vi "hamilton_controller.vi"(8 "error in":errorcluster, 9 "Open?":bool, 10 "valve":enum16{"A", "B", "C", "D", "ALL"}(ring), 11 "action":T1(ring)) -> (0 "error out":errorcluster)   [LabVIEW 2014]
uses:
  <vilib>/Instr/_visa.llb/VISA Configure Serial Port (Instr).vi
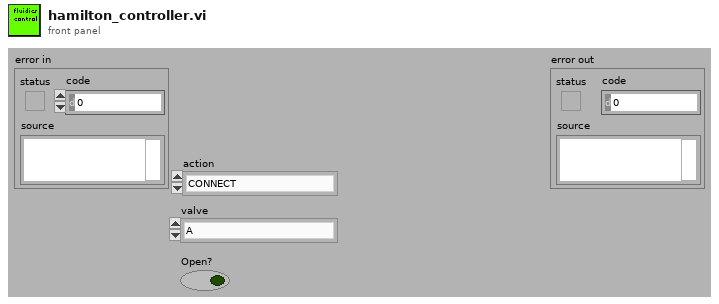
[diagram p1: front panel]
types:
  T1 = enum16{"CONNECT", "INITIALIZE VALVES", "DISCONNECT", "MOVE VALVE"}
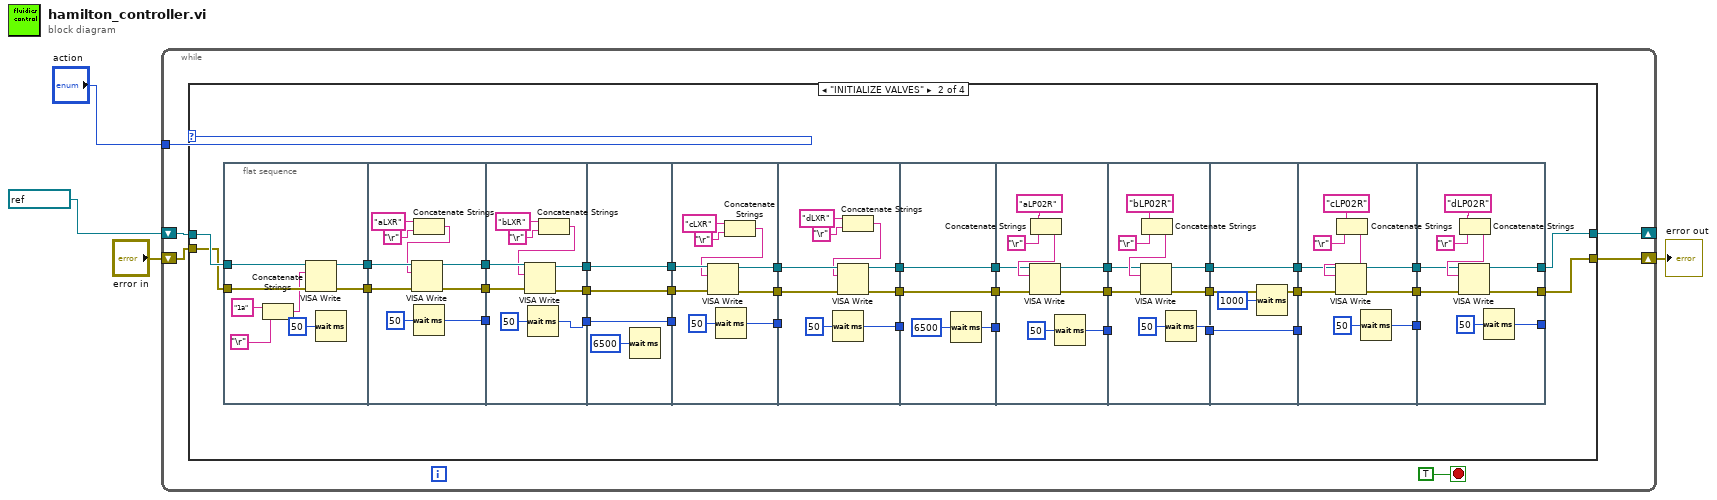
[diagram p0: block diagram]
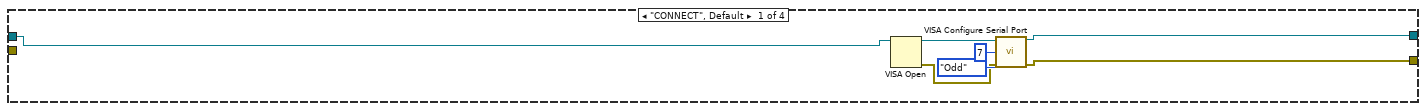
[diagram p2: hidden frame]
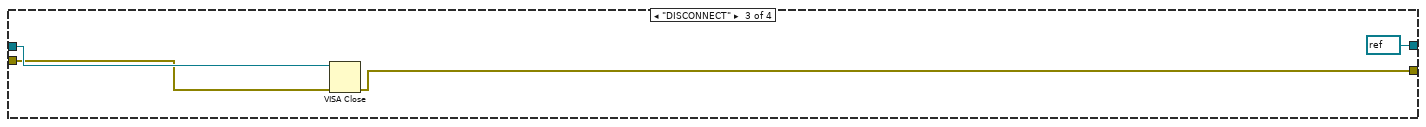
[diagram p3: hidden frame]
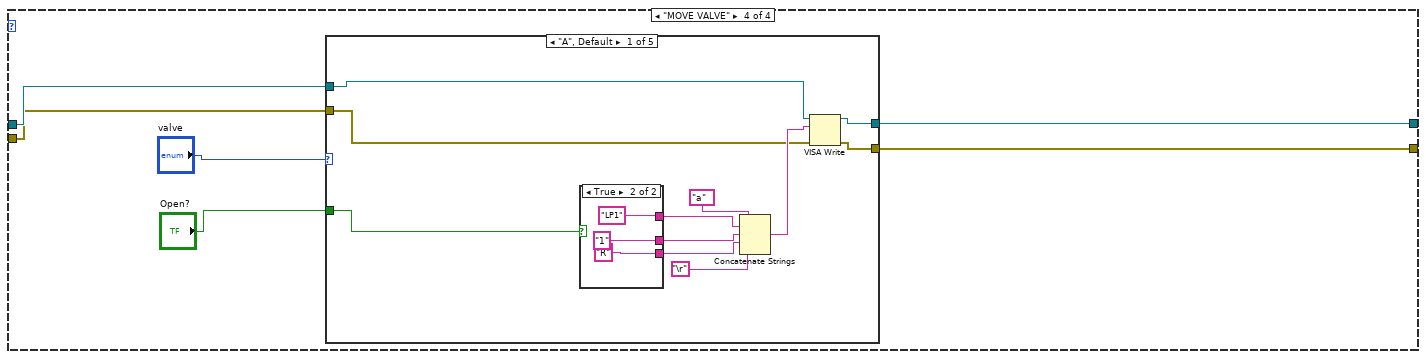
[diagram p4: hidden frame]
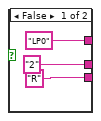
[diagram p5: hidden frame]
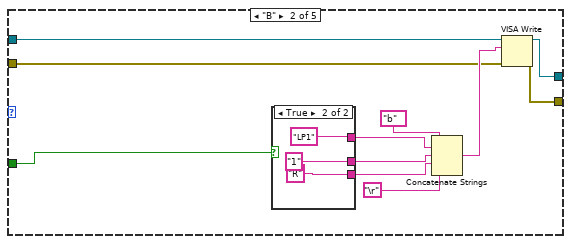
[diagram p6: hidden frame]
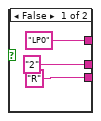
[diagram p7: hidden frame]
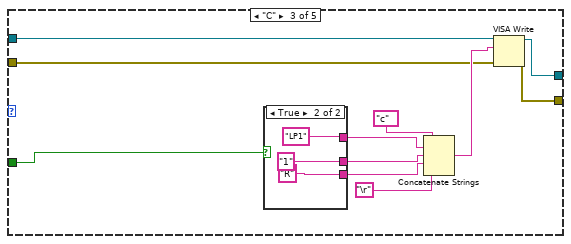
[diagram p8: hidden frame]
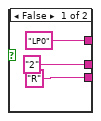
[diagram p9: hidden frame]
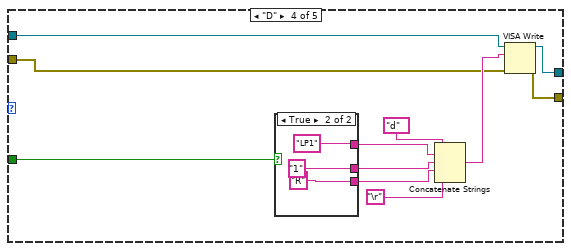
[diagram p10: hidden frame]
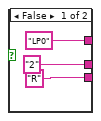
[diagram p11: hidden frame]
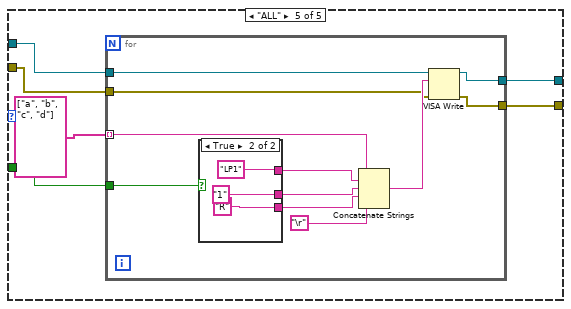
[diagram p12: hidden frame]
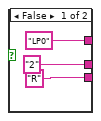
[diagram p13: hidden frame]
diagram:
  n1 = while {
    tunnel: "action" -> [w9]
    shift-right: [w8] -> _
    shift-left: refnum<visa-resource-name> "COM6" ("VISA resource name") -> [w6]
    shift-right: [w7] -> w2
    shift-left: "error in" -> [w5]
    stop <- TRUE stop-if-true
    n2 = case shown="\"INITIALIZE VALVES\"" w9 {
      tunnel: [w13 w19 refnum<visa-resource-name> refnum ("VISA resource name out") w152] -> w8
      tunnel: [w12 w18 w147 w151] -> w7
      tunnel: w6 -> [w11 w21 w149 w154]
      tunnel: w5 -> [_ w20 w148 w153]
      frame "CONNECT", Default {
        n3 = VISA Open(VISA resource name=w11) -> (VISA resource name=w17:refnum<visa-resource-name>, error out=w14:errorcluster)  [unwired: 4 in]
        n4 = call-poly "VISA Configure Serial Port"("VISA resource name"=w17, "data bits (8)"=u16 7, "parity (0:none)"=enum16{"None", "Odd", "Even", "Mark", "Space"}."Odd", "error in (no error)"=w14) -> ("VISA resource name out"=w13:refnum<visa-resource-name>, "error out"=w12:errorcluster)  [unwired: 10 in]
      }
      frame "INITIALIZE VALVES" {
        n5 = flat-sequence {
          tunnel: w21 -> [w61]
          tunnel: w20 -> [w60]
          tunnel: [w59] -> w53
          tunnel: [w55] -> w52
          tunnel: w53 -> [w69]
          tunnel: w52 -> [w70]
          tunnel: [w68] -> w51
          tunnel: [w63] -> w50
          tunnel: [w62] -> w49
          tunnel: w51 -> [_]
          tunnel: w50 -> [w79]
          tunnel: [w78] -> w48
          tunnel: w49 -> [w77]
          tunnel: [w76] -> w47
          tunnel: [w74] -> w46
          tunnel: w48 -> [w83]
          tunnel: [w83] -> w45
          tunnel: w47 -> [w82]
          tunnel: [w82] -> w44
          tunnel: w46 -> [w81]
          tunnel: [w81] -> w43
          tunnel: w45 -> [w92]
          tunnel: [w91] -> w42
          tunnel: w44 -> [w90]
          tunnel: [w89] -> w41
          tunnel: w43 -> [_]
          tunnel: [w87] -> w40
          tunnel: w42 -> [w101]
          tunnel: w41 -> [w100]
          tunnel: w40 -> [_]
          tunnel: [w95] -> w39
          tunnel: [w94] -> w38
          tunnel: [w93] -> w37
          tunnel: w39 -> [w102]
          tunnel: w38 -> [w105]
          tunnel: [w105] -> w36
          tunnel: w37 -> [_]
          tunnel: [w103] -> w35
          tunnel: [w102] -> w34
          tunnel: w36 -> [w108]
          tunnel: w35 -> [_]
          tunnel: w34 -> [w106]
          tunnel: [w111] -> w33
          tunnel: [w109] -> w32
          tunnel: [w107] -> w31
          tunnel: w33 -> [w118]
          tunnel: w32 -> [_]
          tunnel: [w117] -> w30
          tunnel: [w119] -> w29
          tunnel: w31 -> [w116]
          tunnel: [w115] -> w28
          tunnel: w30 -> [w127]
          tunnel: [w127] -> w27
          tunnel: w29 -> [w126]
          tunnel: [w126] -> w26
          tunnel: w28 -> [w125]
          tunnel: [w125] -> w25
          tunnel: w27 -> [w131]
          tunnel: w26 -> [_]
          tunnel: [w132] -> w24
          tunnel: [w130] -> w23
          tunnel: w25 -> [w129]
          tunnel: [w128] -> w22
          tunnel: w24 -> [_]
          tunnel: [w141] -> _
          tunnel: w23 -> [w140]
          tunnel: [w139] -> w18
          tunnel: w22 -> [w138]
          tunnel: [w137] -> w19
          frame #0 {
            n6 = Concatenate Strings("1a" ("string"), "\r") -> (w56:string)
            n7 = VISA Write(VISA resource name=w61, write buffer=w56, error in (no error)=w60) -> (VISA resource name out=w55:refnum<visa-resource-name>, error out=w59:errorcluster)  [unwired: 1 out]
            n8 = Wait (ms)(milliseconds to wait=u32 50) -> ()  [unwired: 1 out]
          }
          frame #1 {
            n9 = Concatenate Strings("aLXR", "\r") -> (w64:string)
            n10 = VISA Write(VISA resource name=w70, write buffer=w64, error in (no error)=w69) -> (VISA resource name out=w63:refnum<visa-resource-name>, error out=w62:errorcluster)  [unwired: 1 out]
            n11 = Wait (ms)(milliseconds to wait=u32 50) -> (millisecond timer value=w68:u32)
          }
          frame #2 {
            n12 = Wait (ms)(milliseconds to wait=u32 50) -> (millisecond timer value=w74:u32)
            n13 = Concatenate Strings("bLXR", "\r") -> (w71:string)
            n14 = VISA Write(VISA resource name=w79, write buffer=w71, error in (no error)=w77) -> (VISA resource name out=w78:refnum<visa-resource-name>, error out=w76:errorcluster)  [unwired: 1 out]
          }
          frame #3 {
            n15 = Wait (ms)(milliseconds to wait=u32 6500) -> ()  [unwired: 1 out]
          }
          frame #4 {
            n16 = Wait (ms)(milliseconds to wait=u32 50) -> (millisecond timer value=w87:u32)
            n17 = Concatenate Strings("cLXR", "\r") -> (w84:string)
            n18 = VISA Write(VISA resource name=w92, write buffer=w84, error in (no error)=w90) -> (VISA resource name out=w91:refnum<visa-resource-name>, error out=w89:errorcluster)  [unwired: 1 out]
          }
          frame #5 {
            n19 = Wait (ms)(milliseconds to wait=u32 50) -> (millisecond timer value=w93:u32)
            n20 = Concatenate Strings("dLXR", "\r") -> (w96:string)
            n21 = VISA Write(VISA resource name=w101, write buffer=w96, error in (no error)=w100) -> (VISA resource name out=w94:refnum<visa-resource-name>, error out=w95:errorcluster)  [unwired: 1 out]
          }
          frame #6 {
            n22 = Wait (ms)(milliseconds to wait=u32 6500) -> (millisecond timer value=w103:u32)
          }
          frame #7 {
            n23 = Concatenate Strings("aLP02R" ("string"), "\r") -> (w114:string)
            n24 = VISA Write(VISA resource name=w108, write buffer=w114, error in (no error)=w106) -> (VISA resource name out=w107:refnum<visa-resource-name>, error out=w111:errorcluster)  [unwired: 1 out]
            n25 = Wait (ms)(milliseconds to wait=u32 50) -> (millisecond timer value=w109:u32)
          }
          frame #8 {
            n26 = Concatenate Strings("bLP02R" ("string"), "\r") -> (w123:string)
            n27 = VISA Write(VISA resource name=w116, write buffer=w123, error in (no error)=w118) -> (VISA resource name out=w115:refnum<visa-resource-name>, error out=w117:errorcluster)  [unwired: 1 out]
            n28 = Wait (ms)(milliseconds to wait=u32 50) -> (millisecond timer value=w119:u32)
          }
          frame #9 {
            n29 = Wait (ms)(milliseconds to wait=u32 1000) -> ()  [unwired: 1 out]
          }
          frame #10 {
            n30 = Concatenate Strings("cLP02R" ("string"), "\r") -> (w136:string)
            n31 = VISA Write(VISA resource name=w129, write buffer=w136, error in (no error)=w131) -> (VISA resource name out=w128:refnum<visa-resource-name>, error out=w130:errorcluster)  [unwired: 1 out]
            n32 = Wait (ms)(milliseconds to wait=u32 50) -> (millisecond timer value=w132:u32)
          }
          frame #11 {
            n33 = Concatenate Strings("dLP02R" ("string"), "\r") -> (w145:string)
            n34 = VISA Write(VISA resource name=w138, write buffer=w145, error in (no error)=w140) -> (VISA resource name out=w137:refnum<visa-resource-name>, error out=w139:errorcluster)  [unwired: 1 out]
            n35 = Wait (ms)(milliseconds to wait=u32 50) -> (millisecond timer value=w141:u32)
          }
        }
      }
      frame "DISCONNECT" {
        n36 = VISA Close(VISA resource name=w149, error in (no error)=w148) -> (error out=w147:errorcluster)
      }
      frame "MOVE VALVE" {
        n37 = case shown="\"A\", Default" "valve" {
          tunnel: w154 -> [w160 w177 w192 w211 w229]
          tunnel: w153 -> [w159 w176 w191 w210 w226]
          tunnel: [w158 w175 w194 w209 w224] -> w152
          tunnel: [w157 w174 w193 w208 w225] -> w151
          tunnel: "Open?" -> [w156 w173 w190 w207 w228]
          frame "A", Default {
            n38 = case shown="True" w156 {
              tunnel: ["R" "R"] -> w164
              tunnel: ["2" "1"] -> w165
              tunnel: ["LP0" ("string") "LP1" ("string")] -> w162
              frame False {
              }
              frame True {
              }
            }
            n39 = Concatenate Strings("a" ("MVP ID"), w162, w165, w164, "\r") -> (w161:string)
            n40 = VISA Write(VISA resource name=w160, write buffer=w161, error in (no error)=w159) -> (VISA resource name out=w158:refnum<visa-resource-name>, error out=w157:errorcluster)  [unwired: 1 out]
          }
          frame "B" {
            n41 = case shown="True" w173 {
              tunnel: ["R" "R"] -> w181
              tunnel: ["2" "1"] -> w182
              tunnel: ["LP0" ("string") "LP1" ("string")] -> w179
              frame False {
              }
              frame True {
              }
            }
            n42 = Concatenate Strings("b" ("MVP ID"), w179, w182, w181, "\r") -> (w178:string)
            n43 = VISA Write(VISA resource name=w177, write buffer=w178, error in (no error)=w176) -> (VISA resource name out=w175:refnum<visa-resource-name>, error out=w174:errorcluster)  [unwired: 1 out]
          }
          frame "C" {
            n44 = case shown="True" w190 {
              tunnel: ["R" "R"] -> w198
              tunnel: ["2" "1"] -> w199
              tunnel: ["LP0" ("string") "LP1" ("string")] -> w196
              frame False {
              }
              frame True {
              }
            }
            n45 = Concatenate Strings("c" ("MVP ID"), w196, w199, w198, "\r") -> (w195:string)
            n46 = VISA Write(VISA resource name=w192, write buffer=w195, error in (no error)=w191) -> (VISA resource name out=w194:refnum<visa-resource-name>, error out=w193:errorcluster)  [unwired: 1 out]
          }
          frame "D" {
            n47 = case shown="True" w207 {
              tunnel: ["R" "R"] -> w215
              tunnel: ["2" "1"] -> w216
              tunnel: ["LP0" ("string") "LP1" ("string")] -> w213
              frame False {
              }
              frame True {
              }
            }
            n48 = Concatenate Strings("d" ("MVP ID"), w213, w216, w215, "\r") -> (w212:string)
            n49 = VISA Write(VISA resource name=w211, write buffer=w212, error in (no error)=w210) -> (VISA resource name out=w209:refnum<visa-resource-name>, error out=w208:errorcluster)  [unwired: 1 out]
          }
          frame "ALL" {
            n50 = for {
              tunnel: w229 -> [w236]
              tunnel: w228 -> [w235]
              tunnel: string[] ["a", "b", "c", "d"] -> [w234] mode=indexing
              tunnel: w226 -> [w232]
              tunnel: [w231] -> w225
              tunnel: [w230] -> w224
              n51 = case shown="True" w235 {
                tunnel: ["R" "R"] -> w239
                tunnel: ["2" "1"] -> w240
                tunnel: ["LP0" ("string") "LP1" ("string")] -> w237
                frame False {
                }
                frame True {
                }
              }
              n52 = Concatenate Strings(w234, w237, w240, w239, "\r") -> (w233:string)
              n53 = VISA Write(VISA resource name=w236, write buffer=w233, error in (no error)=w232) -> (VISA resource name out=w230:refnum<visa-resource-name>, error out=w231:errorcluster)  [unwired: 1 out]
            }
          }
        }
      }
    }
  }
  "error out" <- w2
